vi "Finish.vi"   [LabVIEW 2012]
doc: "This VI is called just before exiting. It is expected to close I/O refnum, save collected data, etc."
uses:
  <vilib>/Rock Robotics/WPI/Compressor/WPI_CompressorGetSetRefNum.vi
  <vilib>/Rock Robotics/WPI/Joystick/WPI_JoystickGetSetRefNum.vi
  <vilib>/Rock Robotics/WPI/RobotDrive/WPI_RobotDriveGetSetRefNum.vi
types:
  T1 = typedef "WPI_DigitalInputDevRef.ctl" = cluster{"DevStatus":errorcluster, "DIO Channel":T2, "Digital Module":T3}
  T2 = typedef "FPGA_DIOChannel.ctl" = enum8{"DIO 1", "DIO 2", "DIO 3", "DIO 4", "DIO 5", "DIO 6", "DIO 7", "DIO 8", "DIO 9", "DIO 10", "DIO 11", "DIO 12", "DIO 13", "DIO 14", "Invalid"}
  T3 = typedef "FPGA_TypedefDigitalModule.ctl" = enum16{"Digital Module 1", "Digital Module 2"}
  T4 = typedef "WPI_EncoderDevRef.ctl" = cluster{"DevStatus":errorcluster, "EncoderIndex":T5, "CounterIndex":T6, "DistancePerCount":dbl, "Decoding Type":T7}
  T5 = typedef "FPGA_EncoderIdx.ctl" = enum8{"Enc 0", "Enc 1", "Enc 2", "Enc 3", "Invalid"}
  T6 = typedef "FPGA_CounterCtrSystemIndex.ctl" = enum8{"Ctr 0", "Ctr 1", "Ctr 2", "Ctr 3", "Ctr 4", "Ctr 5", "Ctr 6", "Ctr 7", "Invalid"}
  T7 = typedef "WPI_EncoderType.ctl" = enum16{"1x", "2x", "4x"}
  T8 = typedef "WPI_CompressorDevRef.ctl" = cluster{"DevStatus":errorcluster, "DigitalInputDevRef":T1, "RelayDevRef":T9}
  T9 = typedef "WPI_RelayDevRef.ctl" = cluster{"DevStatus":errorcluster, "Relay Channel":T10, "Digital Module":T3, "Relay Direction":T11}
  T10 = typedef "FPGA_DIORelayChannel.ctl" = enum8{"Relay 1", "Relay 2", "Relay 3", "Relay 4", "Relay 5", "Relay 6", "Relay 7", "Relay 8", "Invalid"}
  T11 = typedef "WPI_RelayDirection.ctl" = enum16{"Both directions", "Forward only", "Reverse only"}
  T12 = typedef "WPI_RobotDriveDevRef.ctl" = cluster{"DevStatus":errorcluster, "Motors[]":T13[], "Square Inputs":bool, "Max Output":dbl, "Isochronous":bool}
  T13 = typedef "WPI_MotorControlDeviceRef.ctl" = cluster{"DeviceStatus":errorcluster, "Type":enum16{"PWM", "CAN"}, "PWM":cluster{"Digital Module":T3, "PWM Channel":T14, "DeadBand":T15}, "CAN":cluster{"Device Number":u8, "Control Mode":T16, "Semaphore":T17, "Max Vout":dbl}, "Invert":bool, "TransformRef":T18, "InvTransformRef":T18}
  T14 = typedef "FPGA_DIOPWMChannel.ctl" = enum8{"PWM 1", "PWM 2", "PWM 3", "PWM 4", "PWM 5", "PWM 6", "PWM 7", "PWM 8", "PWM 9", "PWM 10", "Invalid"}
  T15 = typedef "WPI_PWMDeadband.ctl" = cluster{"Name":string, "maxPositivePwm":i32, "minPositivePwm":i32, "centerPwm":i32, "maxNegativePwm":i32, "minNegativePwm":i32, "angularRange":u16}
  T16 = typedef "WPI_CANJaguar_ControlMode.ctl" = enum8{"Percent VBus", "Current", "Speed", "Position", "Voltage"}
  T17 = typedef "Semaphore RefNum" = refnum<k1>
  T18 = typedef "WPI_PWMTransform_ConPane.ctl" = refnum<vi>
  T19 = typedef "WPI_JoystickDevRef.ctl" = cluster{"Device":T20}
  T20 = typedef "WPI_JoystickDeviceEnum.ctl" = enum16{"USB 1", "USB 2", "USB 3", "USB 4", "Kinect 1", "Kinect 2"}
  T21 = typedef "WPI_AnalogChannelDevRef.ctl" = cluster{"DevStatus":errorcluster, "Analog Module":T22, "Analog Channel":T23}
  T22 = typedef "FPGA_TypedefAnalogModule.ctl" = enum16{"Analog Module 1", "Analog Module 2"}
  T23 = typedef "FPGA_AIChannel.ctl" = enum8{"AI 1", "AI 2", "AI 3", "AI 4", "AI 5", "AI 6", "AI 7", "AI 8", "Invalid"}
  T24 = typedef "WPI_SolenoidDevRef.ctl" = cluster{"DevStatus":errorcluster, "Solenoid Module":T25, "Forward Solenoid Channel":T26, "Reverse Solenoid Channel":T26}
  T25 = typedef "FPGA_TypedefSolenoidModule.ctl" = enum16{"Solenoid Module 1", "Solenoid Module 2"}
  T26 = typedef "WPI_SolenoidChannel.ctl" = enum8{"Solenoid 1", "Solenoid 2", "Solenoid 3", "Solenoid 4", "Solenoid 5", "Solenoid 6", "Solenoid 7", "Solenoid 8", "Invalid"}
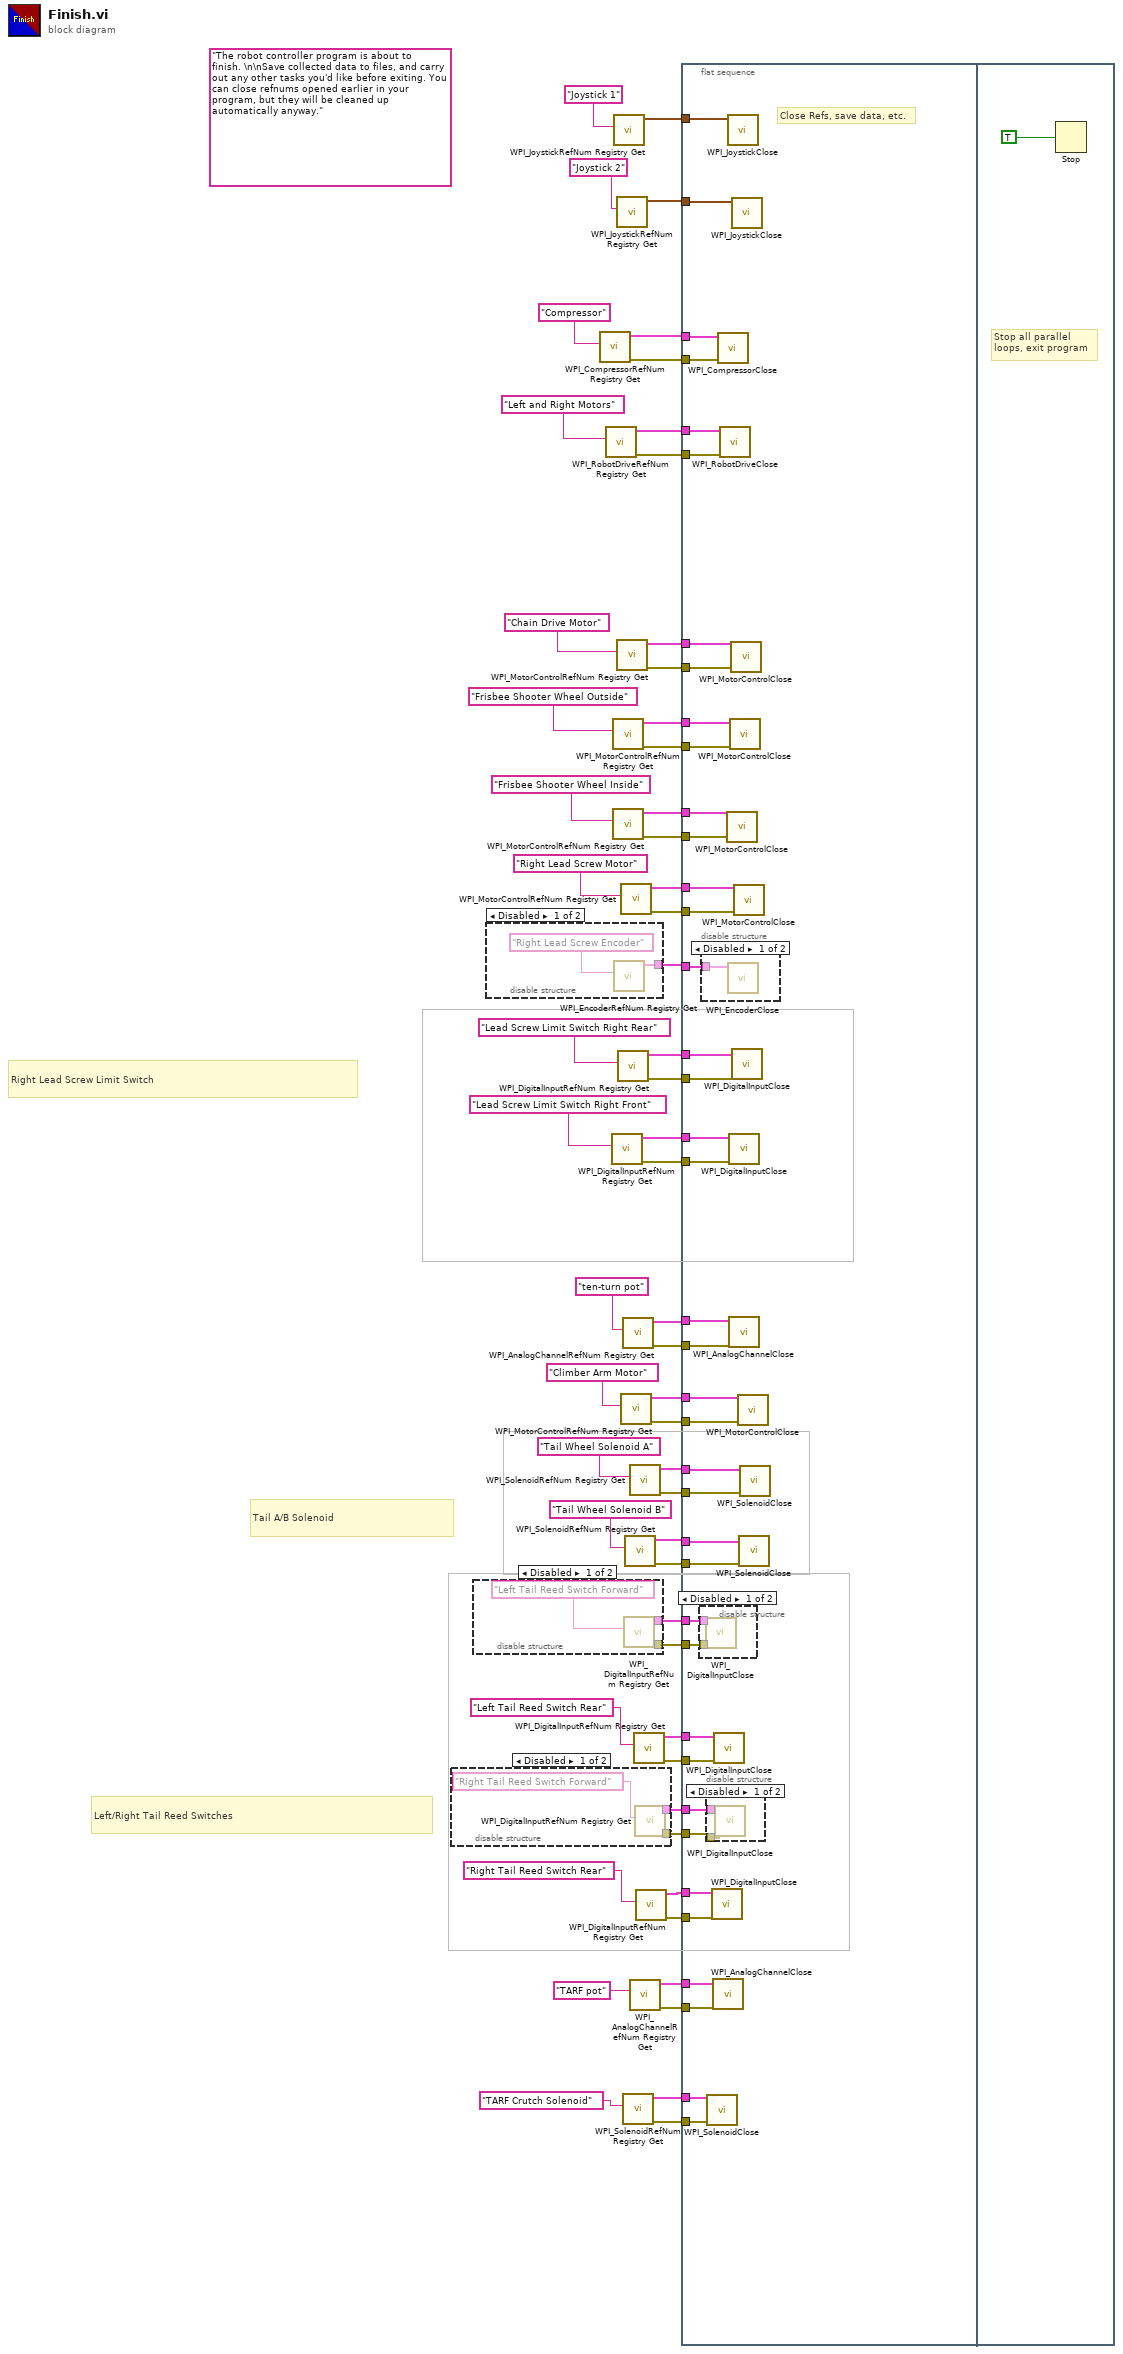
[diagram p0: block diagram]
diagram:
  (unwired) "The robot controller program is about to finish. \n\nSave collected data to files, and carry out any other tasks you'd like before exiting. You can close refnums opened earlier in your program, but they will be cleaned up automatically anyway."
  # "Right Lead Screw Limit Switch"
  # "Tail A/B Solenoid"
  # "Left/Right Tail Reed Switches"
  n1 = disable-structure shown="Disabled" {
    disable-tunnel: [w60 _] -> w27
    disable-tunnel: [w58 _] -> w17
    frame Disabled {
      n2 = call <vilib>:"WPI_DigitalInputRefNum Registry Get.vi"("refnum name"="Right Tail Reed Switch Forward") -> ("error out"=w58:errorcluster, "DigitalInputDevRef"=w60:T1)  [unwired: 9 in]
    }
    frame Enabled {
    }
  }
  n3 = disable-structure shown="Disabled" {
    disable-tunnel: [w62 _] -> w29
    disable-tunnel: [w61 _] -> w16
    frame Disabled {
      n4 = call <vilib>:"WPI_DigitalInputRefNum Registry Get.vi"("refnum name"="Left Tail Reed Switch Forward") -> ("error out"=w61:errorcluster, "DigitalInputDevRef"=w62:T1)  [unwired: 9 in]
    }
    frame Enabled {
    }
  }
  n5 = disable-structure shown="Disabled" {
    disable-tunnel: [w65 _] -> w42
    frame Disabled {
      n6 = call <vilib>:"WPI_EncoderRefNum Registry Get.vi"("refnum name"="Right Lead Screw Encoder") -> ("EncoderDevRef"=w65:T4)  [unwired: 9 in, 1 out]
    }
    frame Enabled {
    }
  }
  n7 = call <vilib>:"WPI_CompressorRefNum Registry Get.vi"("refnum name"="Compressor") -> ("error out"=w4:errorcluster, "CompressorDevRef"=w23:T8)  [unwired: 9 in]
  n8 = call <vilib>:"WPI_RobotDriveRefNum Registry Get.vi"("refnum name"="Left and Right Motors") -> ("error out"=w5:errorcluster, "RobotDriveDevRef"=w55:T12)  [unwired: 1 in, 8 out]
  n9 = call <vilib>:"WPI_DigitalInputRefNum Registry Get.vi"("refnum name"="Lead Screw Limit Switch Right Front") -> ("error out"=w11:errorcluster, "DigitalInputDevRef"=w38:T1)  [unwired: 9 in]
  n10 = call <vilib>:"WPI_MotorControlRefNum Registry Get.vi"("refnum name"="Frisbee Shooter Wheel Outside") -> ("error out"=w7:errorcluster, "MotorControlDevRef"=w46:T13)  [unwired: 9 in]
  n11 = call <vilib>:"WPI_MotorControlRefNum Registry Get.vi"("refnum name"="Frisbee Shooter Wheel Inside") -> ("error out"=w8:errorcluster, "MotorControlDevRef"=w45:T13)  [unwired: 9 in]
  n12 = call <vilib>:"WPI_JoystickRefNum Registry Get.vi"("refnum name"="Joystick 1") -> ("JoystickDevRef"=w54:T19)  [unwired: 1 in, 9 out]
  n13 = call <vilib>:"WPI_JoystickRefNum Registry Get.vi"("refnum name"="Joystick 2") -> ("JoystickDevRef"=w52:T19)  [unwired: 1 in, 9 out]
  n14 = call <vilib>:"WPI_MotorControlRefNum Registry Get.vi"("refnum name"="Chain Drive Motor") -> ("error out"=w6:errorcluster, "MotorControlDevRef"=w47:T13)  [unwired: 9 in]
  n15 = call <vilib>:"WPI_DigitalInputRefNum Registry Get.vi"("refnum name"="Lead Screw Limit Switch Right Rear") -> ("error out"=w10:errorcluster, "DigitalInputDevRef"=w39:T1)  [unwired: 9 in]
  n16 = call <vilib>:"WPI_MotorControlRefNum Registry Get.vi"("refnum name"="Right Lead Screw Motor") -> ("error out"=w9:errorcluster, "MotorControlDevRef"=w44:T13)  [unwired: 9 in]
  n17 = call <vilib>:"WPI_MotorControlRefNum Registry Get.vi"("refnum name"="Climber Arm Motor") -> ("error out"=w13:errorcluster, "MotorControlDevRef"=w34:T13)  [unwired: 9 in]
  n18 = call <vilib>:"WPI_AnalogChannelRefNum Registry Get.vi"("refnum name"="ten-turn pot") -> ("error out"=w12:errorcluster, "AIDeviceRef"=w36:T21)  [unwired: 9 in]
  n19 = call <vilib>:"WPI_SolenoidRefNum Registry Get.vi"("refnum name"="TARF Crutch Solenoid") -> ("error out"=w2:errorcluster, "SolenoidDevRef"=w3:T24)  [unwired: 9 in]
  n20 = call <vilib>:"WPI_SolenoidRefNum Registry Get.vi"("refnum name"="Tail Wheel Solenoid B") -> ("error out"=w15:errorcluster, "SolenoidDevRef"=w30:T24)  [unwired: 9 in]
  n21 = call <vilib>:"WPI_SolenoidRefNum Registry Get.vi"("refnum name"="Tail Wheel Solenoid A") -> ("error out"=w14:errorcluster, "SolenoidDevRef"=w31:T24)  [unwired: 9 in]
  n22 = call <vilib>:"WPI_AnalogChannelRefNum Registry Get.vi"("refnum name"="TARF pot") -> ("error out"=w20:errorcluster, "AIDeviceRef"=w21:T21)  [unwired: 9 in]
  n23 = call <vilib>:"WPI_DigitalInputRefNum Registry Get.vi"("refnum name"="Left Tail Reed Switch Rear") -> ("error out"=w18:errorcluster, "DigitalInputDevRef"=w28:T1)  [unwired: 9 in]
  n24 = call <vilib>:"WPI_DigitalInputRefNum Registry Get.vi"("refnum name"="Right Tail Reed Switch Rear") -> ("error out"=w19:errorcluster, "DigitalInputDevRef"=w26:T1)  [unwired: 9 in]
  n25 = flat-sequence {
    tunnel: w55 -> [w104]
    tunnel: w54 -> [w103]
    tunnel: w52 -> [w102]
    tunnel: w23 -> [w101]
    tunnel: w47 -> [w100]
    tunnel: w46 -> [w99]
    tunnel: w45 -> [w98]
    tunnel: w44 -> [w97]
    tunnel: w42 -> [w96]
    tunnel: w39 -> [w95]
    tunnel: w38 -> [w94]
    tunnel: w36 -> [w93]
    tunnel: w34 -> [w92]
    tunnel: w31 -> [w91]
    tunnel: w30 -> [w90]
    tunnel: w29 -> [w89]
    tunnel: w28 -> [w88]
    tunnel: w27 -> [w87]
    tunnel: w26 -> [w86]
    tunnel: w21 -> [w85]
    tunnel: w20 -> [w84]
    tunnel: w19 -> [w83]
    tunnel: w18 -> [w82]
    tunnel: w17 -> [w81]
    tunnel: w16 -> [w80]
    tunnel: w15 -> [w79]
    tunnel: w14 -> [w78]
    tunnel: w13 -> [w77]
    tunnel: w12 -> [w76]
    tunnel: w11 -> [w75]
    tunnel: w10 -> [w74]
    tunnel: w9 -> [w73]
    tunnel: w8 -> [w72]
    tunnel: w7 -> [w71]
    tunnel: w6 -> [w70]
    tunnel: w5 -> [w69]
    tunnel: w4 -> [w68]
    tunnel: w3 -> [w67]
    tunnel: w2 -> [w66]
    frame #0 {
      # "Close Refs, save data, etc."
      n26 = disable-structure shown="Disabled" {
        disable-tunnel: w89 -> [w108 _]
        disable-tunnel: w80 -> [_ _]
        frame Disabled {
          n27 = call <vilib>:"WPI_DigitalInputClose.vi"("DigitalInputDevRef"=w108) -> ()  [unwired: 10 in, 1 out]
        }
        frame Enabled {
        }
      }
      n28 = disable-structure shown="Disabled" {
        disable-tunnel: w96 -> [w105 _]
        frame Disabled {
          n29 = call <vilib>:"WPI_EncoderClose.vi"("EncoderDevRef"=w105) -> ()  [unwired: 10 in, 1 out]
        }
        frame Enabled {
        }
      }
      n30 = disable-structure shown="Disabled" {
        disable-tunnel: w87 -> [w107 _]
        disable-tunnel: w81 -> [w106 _]
        frame Disabled {
          n31 = call <vilib>:"WPI_DigitalInputClose.vi"("error in (no error)"=w106, "DigitalInputDevRef"=w107) -> ()  [unwired: 9 in, 1 out]
        }
        frame Enabled {
        }
      }
      n32 = call <vilib>:"WPI_SolenoidClose.vi"("error in (no error)"=w66, "SolenoidDevRef"=w67) -> ()  [unwired: 9 in, 1 out]
      n33 = call <vilib>:"WPI_DigitalInputClose.vi"("error in (no error)"=w83, "DigitalInputDevRef"=w86) -> ()  [unwired: 9 in, 1 out]
      n34 = call <vilib>:"WPI_AnalogChannelClose.vi"("error in (no error)"=w84, "AIDeviceRef"=w85) -> ()  [unwired: 9 in, 1 out]
      n35 = call <vilib>:"WPI_DigitalInputClose.vi"("error in (no error)"=w82, "DigitalInputDevRef"=w88) -> ()  [unwired: 9 in, 1 out]
      n36 = call <vilib>:"WPI_CompressorClose.vi"("error in (no error)"=w68, "CompressorDevRef"=w101) -> ()  [unwired: 9 in, 1 out]
      n37 = call <vilib>:"WPI_RobotDriveClose.vi"("error in (no error)"=w69, "RobotDriveDevRef"=w104) -> ()  [unwired: 10 out]
      n38 = call <vilib>:"WPI_MotorControlClose.vi"("error in (no error)"=w72, "MotorControlDevRef"=w98) -> ()  [unwired: 9 in, 1 out]
      n39 = call <vilib>:"WPI_JoystickClose.vi"("JoystickDevRef"=w103) -> ()  [unwired: 11 out]
      n40 = call <vilib>:"WPI_DigitalInputClose.vi"("error in (no error)"=w75, "DigitalInputDevRef"=w94) -> ()  [unwired: 9 in, 1 out]
      n41 = call <vilib>:"WPI_AnalogChannelClose.vi"("error in (no error)"=w76, "AIDeviceRef"=w93) -> ()  [unwired: 9 in, 1 out]
      n42 = call <vilib>:"WPI_MotorControlClose.vi"("error in (no error)"=w71, "MotorControlDevRef"=w99) -> ()  [unwired: 9 in, 1 out]
      n43 = call <vilib>:"WPI_MotorControlClose.vi"("error in (no error)"=w70, "MotorControlDevRef"=w100) -> ()  [unwired: 9 in, 1 out]
      n44 = call <vilib>:"WPI_JoystickClose.vi"("JoystickDevRef"=w102) -> ()  [unwired: 11 out]
      n45 = call <vilib>:"WPI_DigitalInputClose.vi"("error in (no error)"=w74, "DigitalInputDevRef"=w95) -> ()  [unwired: 9 in, 1 out]
      n46 = call <vilib>:"WPI_MotorControlClose.vi"("error in (no error)"=w73, "MotorControlDevRef"=w97) -> ()  [unwired: 9 in, 1 out]
      n47 = call <vilib>:"WPI_MotorControlClose.vi"("error in (no error)"=w77, "MotorControlDevRef"=w92) -> ()  [unwired: 9 in, 1 out]
      n48 = call <vilib>:"WPI_SolenoidClose.vi"("error in (no error)"=w79, "SolenoidDevRef"=w90) -> ()  [unwired: 9 in, 1 out]
      n49 = call <vilib>:"WPI_SolenoidClose.vi"("error in (no error)"=w78, "SolenoidDevRef"=w91) -> ()  [unwired: 9 in, 1 out]
    }
    frame #1 {
      # "Stop all parallel\nloops, exit program"
      n50 = Stop(stop? (T)=TRUE ("Quit")) -> ()
    }
  }
